vi "Add ColumHead Items by Text Array.vi"(8 "error in (no error)":errorcluster caption="错误输入（无错误）", 10 "Text":string[](array[string]), 11 "ListViewClass 输入":refnum<class "ListViewClass.lvclass"> caption="DNL_LabVIEW Object in") -> (0 "error out":errorcluster caption="错误输出", 3 "ListViewClass 输出":refnum<class "ListViewClass.lvclass"> caption="DNL_LabVIEW Object out")   [LabVIEW 2012, in "ListViewClass.lvclass"]
uses:
  ListViewClass.lvclass
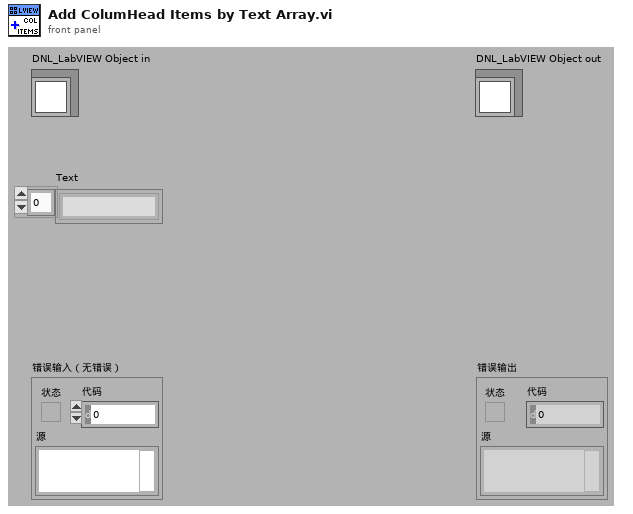
[diagram p1: front panel]
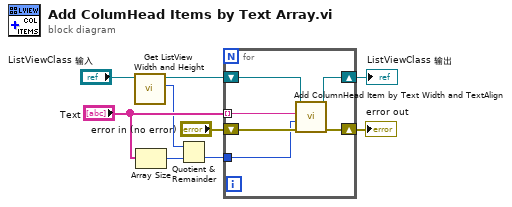
[diagram p0: block diagram]
diagram:
  n1 = call "Get ListView Width and Height.vi"("ListViewClass 输入"="ListViewClass 输入") -> ("Width"=w3:i32, "ListViewClass 输出"=w5:refnum<class "ListViewClass.lvclass">)  [unwired: 7 in, 2 out]
  n2 = Array Size(array="Text") -> (size(s)=w2:i32)
  n3 = Quotient & Remainder(x=w3, y=w2) -> (floor(x/y)=w1:i32)  [unwired: 1 out]
  n4 = for {
    shift-right: [w14] -> w9
    shift-left: w5 -> [w15]
    shift-right: [w12] -> w7
    shift-left: "error in (no error)" -> [w13]
    tunnel: "Text" -> [w11] mode=indexing
    tunnel: w1 -> [w10]
    n5 = call "Add ColumnHead Item by Text Width and TextAlign.vi"("error in (no error)"=w13, "width"=w10, "text"=w11, "ListViewClass 输入"=w15) -> ("error out"=w12:errorcluster, "ListViewClass 输出"=w14:refnum<class "ListViewClass.lvclass">)  [unwired: 6 in]
  }
  "error out" <- w7
  "ListViewClass 输出" <- w9
